vi "ME103 Lab1B SP26.vi"() -> ()   [LabVIEW 2025]
panel:
  in  "Data Stream":bool
  out "Fan Voltage":dbl caption="Volts"
  in  "Stop VI":bool
  out "IR Sensor Voltage":dbl caption="Volts"
  # "Part 3 - Ping Pong Tower Experimentation"
  # "Use this LabVIEW VI to monitor the voltage output from the IR sensor, and the voltage draw from the fan.\n\nAfter you start/run this VI, click on the Data Stream button (green circle should light up) to start reading the voltages. Click it again to pause reading the voltages. Clicking the Data Stream button after that will resume the voltage reading.  \n\nDo this as many times as you want when monitoring the behavior of the ping pong tower. When you are finished click on the Stop VI Program button."
  # "ME 103 Experimentation and Measurements"
  # "Lab 1 Part 3: Ping Pong Tower Experimentation"
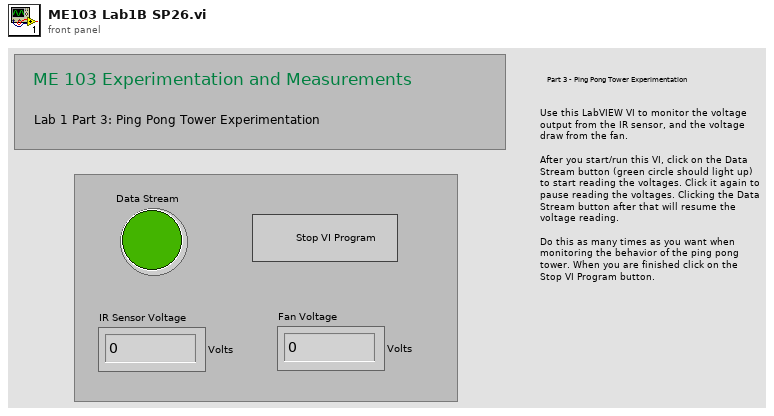
[diagram p1: front panel]
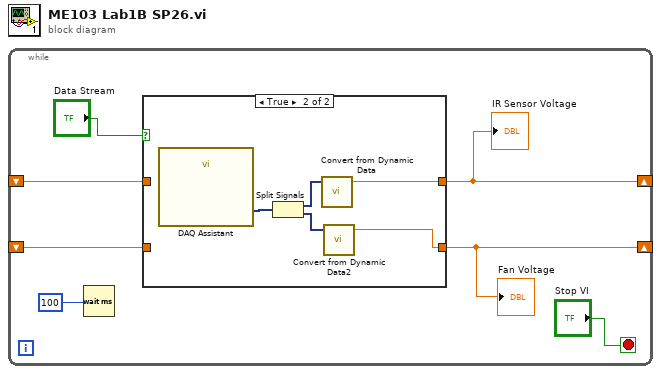
[diagram p0: block diagram]
diagram:
  n1 = while {
    shift-right: [w7] -> _
    shift-left: _ -> [w6]
    shift-right: [w1] -> _
    shift-left: _ -> [w3]
    stop <- "Stop VI" stop-if-true
    n2 = Wait (ms)(milliseconds to wait=u32 100) -> ()  [unwired: 1 out]
    n3 = case shown="True" "Data Stream" {
      tunnel: [w9 w14] -> w7
      tunnel: w6 -> [w9 _]
      tunnel: [w8 w10] -> w1
      tunnel: w3 -> [w8 _]
      frame False {
      }
      frame True {
        n4 = call "DAQ Assistant"() -> ("data"=w13:dynamicdata)  [unwired: 17 in, 2 out]
        n5 = Split Signals(w13) -> (w12:dynamicdata, w11:dynamicdata)  [unwired: 2 in]
        n6 = call "Convert from Dynamic Data"("Dynamic Data Type"=w12) -> ("Scalar"=w14:dbl)  [unwired: 3 in]
        n7 = call "Convert from Dynamic Data2"("Dynamic Data Type"=w11) -> ("Scalar"=w10:dbl)  [unwired: 3 in]
      }
    }
    "IR Sensor Voltage" <- w7
    "Fan Voltage" <- w1
  }
